vi "TSM Relay Close Sessions.vi"(0 "TSM context":T1) -> (15 "error out":errorcluster)   [LabVIEW 2020]
doc: "Use this VI to reset and close all sessions for all NI-RELAY (Switch) instruments in the Semiconductor Module Context."
uses:
  <vilib>/NI_TestStand_SemiconductorModule/NI_TestStand_Semiconductor_Module.lvlibp/PinMap/General/SemiconductorModuleContext.ctl
  <vilib>/NI_TestStand_SemiconductorModule/NI_TestStand_Semiconductor_Module.lvlibp
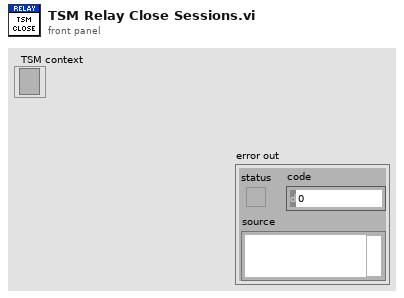
[diagram p1: front panel]
types:
  T1 = typedef "NI_TestStand_Semiconductor_Module.lvlibp/SemiconductorModuleContext.ctl" = refnum<k7>
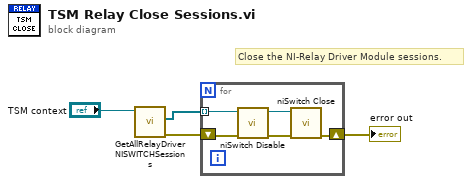
[diagram p0: block diagram]
diagram:
  # "Close the NI-Relay Driver Module sessions."
  n1 = call <vilib>:"GetAllRelayDriverNISWITCHSessions.vi"("Semiconductor Module Context"="TSM context") -> ("error out"=w2:errorcluster, "NI-SWITCH Sessions"=w1:refnum<k15>[])  [unwired: 8 in, 1 out]
  n2 = for {
    tunnel: w1 -> [w6] mode=indexing
    shift-right: [w9] -> w4
    shift-left: w2 -> [w8]
    n3 = call <instrlib>:"niSwitch Disable.vi"("error in (no error)"=w8, "instrument handle"=w6) -> ("error out"=w7:errorcluster, "instrument handle out"=w5:refnum<k15>)  [unwired: 8 in]
    n4 = call <instrlib>:"niSwitch Close.vi"("error in (no error)"=w7, "instrument handle"=w5) -> ("error out"=w9:errorcluster)  [unwired: 9 in]
  }
  "error out" <- w4
